vi "Create Panel by Type.vi"(7 "Panel Type":refnum<class "ArrayPanel.lvclass">, 8 "error in (no error)":errorcluster, 9 "Run? (T)":bool=TRUE, 11 "2DArrayManager in":refnum<class "2DArrayManager.lvclass">) -> (0 "error out":errorcluster, 2 "Panel":refnum<class "ArrayPanel.lvclass">, 3 "2DArrayManager out":refnum<class "2DArrayManager.lvclass">)   [LabVIEW 2020, in "OOPanel.lvlib" / "2DArrayManager.lvclass"]
uses:
  2DArrayManager.lvclass
  2DArrayManager.lvclass/2DArrayManager.ctl
  Manager/Manager.lvclass
  ArrayPanel/ArrayPanel.lvclass
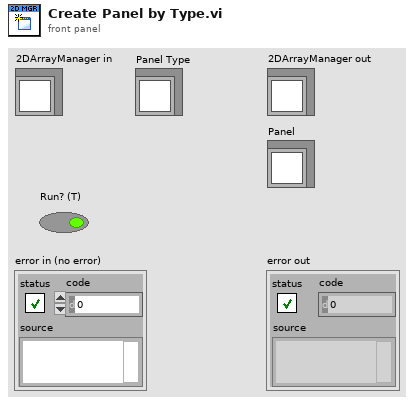
[diagram p1: front panel]
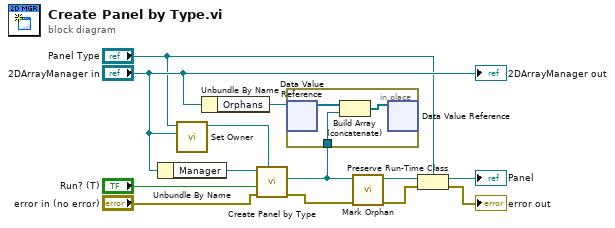
[diagram p0: block diagram]
diagram:
  n1 = Unbundle By Name("2DArrayManager in") -> ("Manager"=w13:refnum<class "Manager.lvclass">)
  n2 = call "Set Owner.vi"("Owner"="2DArrayManager in", "ArrayPanel in"="Panel Type") -> ("ArrayPanel out"=w12:refnum<class "ArrayPanel.lvclass">)  [unwired: 8 in, 1 out]
  n3 = Unbundle By Name("2DArrayManager in") -> ("Orphans"=w10:refnum<data-value>)
  n4 = call "Create Panel by Type.vi"("Panel Type"=w12, "error in (no error)"="error in (no error)", "Run? (T)"="Run? (T)", "Manager in"=w13) -> ("error out"=w7:errorcluster, "Panel"=w4:refnum<class "ArrayPanel.lvclass">)  [unwired: 5 in, 1 out]
  n5 = in-place {
    in-place-border: w4 -> [w15]
    n6 = in-place-dvr #1(w10) -> (w16:refnum<class "ArrayPanel.lvclass">[])  [unwired: 1 out]
    n7 = Build Array (concatenate)(w16, w15) -> (w14:refnum<class "ArrayPanel.lvclass">[])
    n8 = in-place-dvr #1(w14) -> ()  [unwired: 2 out]
  }
  n9 = call "Mark Orphan.vi"("error in (no error)"=w7, "ArrayPanel in"=w4) -> ("error out"=w6:errorcluster, "ArrayPanel out"=w2:refnum<class "ArrayPanel.lvclass">)  [unwired: 8 in]
  n10 = Preserve Run-Time Class(object in=w2, error in=w6, 2:"Panel Type") -> (object out=→"Panel":refnum<class "ArrayPanel.lvclass">, error out=→"error out":errorcluster)
  "2DArrayManager out" <- "2DArrayManager in"
